vi "wait on clock.vi"(8 "error in":errorcluster, 10 "dt":u32=1, 11 "timing source in":refnum<class "usec timing source.lvclass">) -> (0 "error out":errorcluster, 2 "ticks since last call":u32, 3 "timing source out":refnum<class "usec timing source.lvclass">)   [LabVIEW 2013, in "usec timing source.lvclass"]
doc: "This core timing function is used inside of a loop to wait for a clock signal, or dt ticks of a clock signal."
uses:
  usec timing source.lvclass
  usec timing source.lvclass/usec timing source.ctl
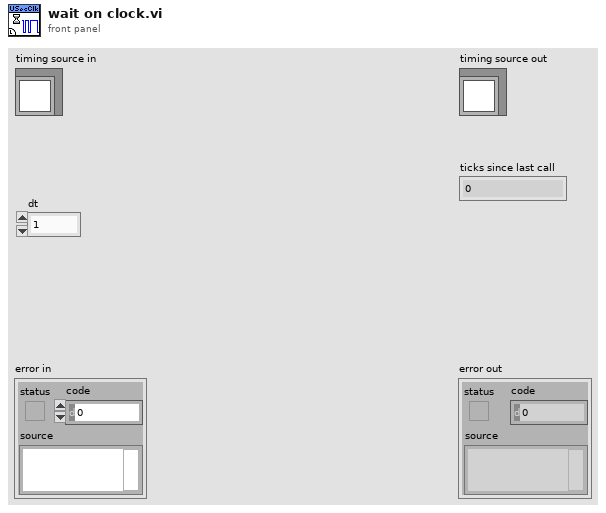
[diagram p1: front panel]
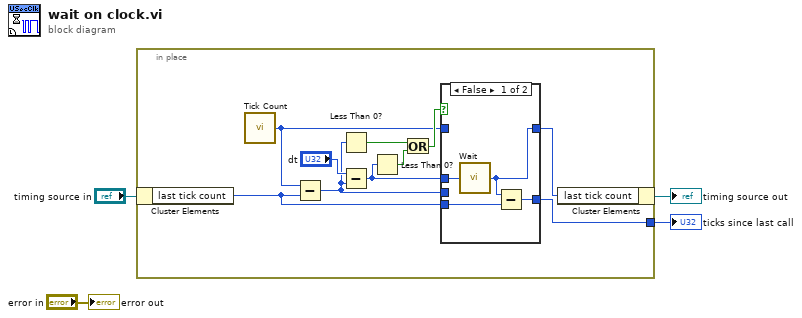
[diagram p0: block diagram]
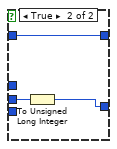
[diagram p2: hidden frame]
diagram:
  n1 = in-place {
    in-place-border: [w8] -> w1
    n2 = in-place-cluster #1("timing source in") -> ("last tick count"=w5:u32)
    n3 = call "Tick Count"() -> ("Tick Count(uSec)"=w9:u32)
    n4 = Subtract(x=w9, y=w5) -> (x-y=w7:i64)
    n5 = Less Than 0?(x=w7) -> (x < 0?=w12:bool)
    n6 = Subtract(x="dt", y=w7) -> (x-y=w6:i64)
    n7 = Less Than 0?(x=w6) -> (x < 0?=w13:bool)
    n8 = Or(x=w12, y=w13) -> (x .or. y?=w11:bool)
    n9 = case shown="False" w11 {
      tunnel: [w17 w21] -> w10
      tunnel: w9 -> [_ w21]
      tunnel: [w16 w19] -> w8
      tunnel: w7 -> [_ w20]
      tunnel: w6 -> [w18 _]
      tunnel: w5 -> [w15 _]
      frame False {
        n10 = call "Wait"("Count(uSec)"=w18) -> ("Tick Count(uSec)"=w17:u32)
        n11 = Subtract(x=w17, y=w15) -> (x-y=w16:u32)
      }
      frame True {
        n12 = To Unsigned Long Integer(number=w20) -> (unsigned 32bit integer=w19:u32)
      }
    }
    n13 = in-place-cluster #1("last tick count"=w10) -> (→"timing source out":refnum<class "usec timing source.lvclass">)
  }
  "ticks since last call" <- w1
  "error out" <- "error in"
